vi "日期字符串格式至时间格式转换(子VI).vi"(11 "data[0]":string) -> (3 "time stamp":timestamp format="%<%Y/%m/%d %H:%M:%S>T")   [LabVIEW 2016]
uses:
  <vilib>/Utility/miscctls.llb/LVDateTimeRec.ctl
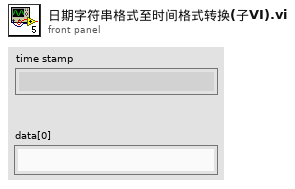
[diagram p1: front panel]
types:
  T1 = typedef "LVDateTimeRec.ctl" = cluster{"fractional second":dbl, "second":i32, "minute":i32, "hour":i32, "day of month":i32, "month":i32, "year":i32, "day of week":i32, "day of year":i32, "DST":i32}
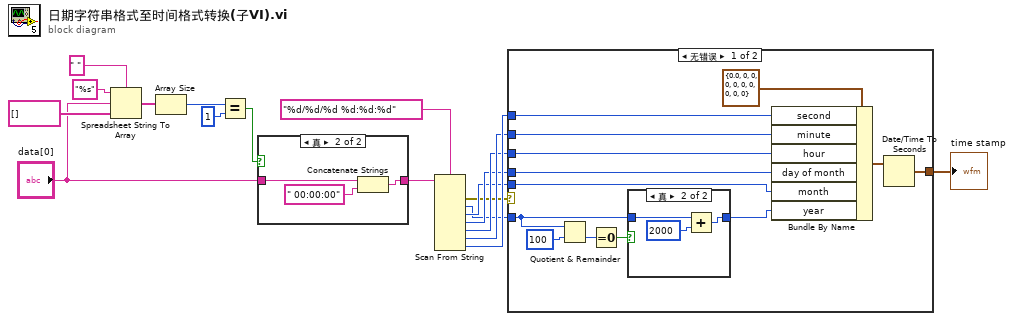
[diagram p0: block diagram]
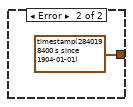
[diagram p4: hidden frame]
diagram:
  n1 = Spreadsheet String To Array(delimiter (Tab)=" " ("分隔符(Tab)"), format string="%s" ("格式字符串"), spreadsheet string="data[0]", array type (2D Dbl)=string[] []) -> (array=w6:string[])
  n2 = Array Size(array=w6) -> (size(s)=w5:i32)
  n3 = Equal?(x=w5, y=1) -> (x = y?=w3:bool)
  n4 = case shown="真" w3 {
    tunnel: "data[0]" -> [w19 w21]
    tunnel: [w19 w20] -> w1
    frame False {
    }
    frame True {
      n5 = Concatenate Strings(w21, " 00:00:00" ("字符串")) -> (w20:string)
    }
  }
  n6 = Scan From String(format string="%d/%d/%d %d:%d:%d" ("格式字符串"), input string=w1) -> (error out=w11:errorcluster, output 1=w13:i32, output 2=w14:i32, output 3=w15:i32, output 4=w16:i32, output 5=w17:i32, output 6=w18:i32)  [unwired: 8 in, 2 out]
  n7 = case shown="无错误" w11 {
    tunnel: w18 -> [w34 _]
    tunnel: w17 -> [w33 _]
    tunnel: w16 -> [w32 _]
    tunnel: w15 -> [w31 _]
    tunnel: w14 -> [w30 _]
    tunnel: w13 -> [w26 _]
    tunnel: [w28 timestamp(2840198400 s since 1904-01-01) ("time stamp")] -> w10
    frame No Error {
      n8 = Quotient & Remainder(x=w26, y=100) -> (floor(x/y)=w25:i32)  [unwired: 1 out]
      n9 = Equal To 0?(x=w25) -> (x = 0?=w24:bool)
      n10 = case shown="真" w24 {
        tunnel: w26 -> [w36 w39]
        tunnel: [w36 w37] -> w23
        frame False {
        }
        frame True {
          n11 = Add(x=w39, y=2000) -> (x+y=w37:i32)
        }
      }
      n12 = Bundle By Name(cluster=T1 {"fractional second"=0.0, "second"=0, "minute"=0, "hour"=0, "day of month"=0, "month"=0, "year"=0, "day of week"=0, "day of year"=0, "DST"=0} ("日期时间记录"), "second"=w34, "minute"=w33, "hour"=w32, "day of month"=w31, "month"=w30, "year"=w23) -> (w35:T1)
      n13 = Date/Time To Seconds(2:w35) -> (0:w28:timestamp)  [unwired: 1 in]
    }
    frame Error {
    }
  }
  "time stamp" <- w10
